vi "Create.vi"(0 "vi reference":refnum<vi>, 5 "Ctrl Sequences":string[](array[string]), 11 "error in (no error)":errorcluster) -> (4 "vi reference out":refnum<vi>, 6 "Connector Pane Type":T1, 15 "error out":errorcluster)   [LabVIEW 2018, in "NISAST VI Scripting.lvlib" / "VI.lvlib" / "Connector.lvlib"]
uses:
  Connector.lvlib
  Front Panel/Attribute/Connector Pane Type.ctl
  Front Panel/Front Panel.lvlib
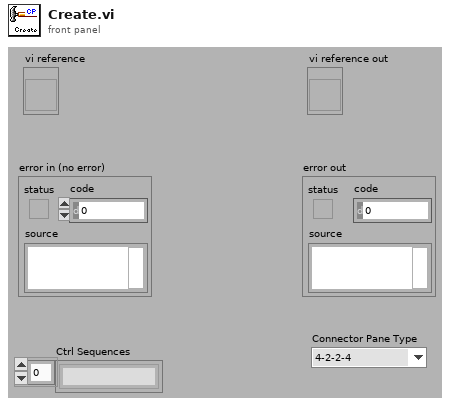
[diagram p1: front panel]
types:
  T1 = typedef "NISAST VI Scripting.lvlib/VI.lvlib/Front Panel.lvlib/Connector Pane Type.ctl" = enum16{"4-2-2-4", "5-2-2-2-5", "Others"}
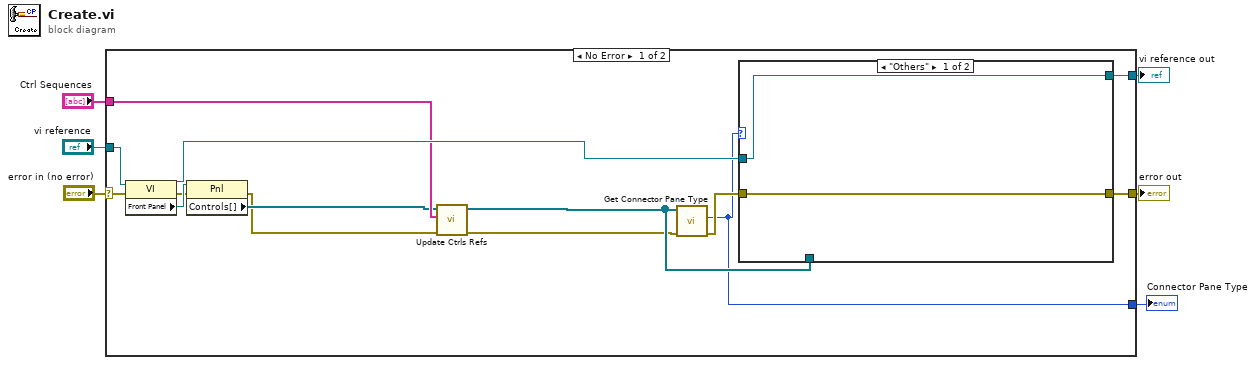
[diagram p0: block diagram]
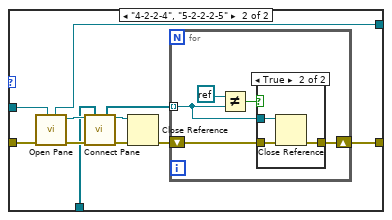
[diagram p2: hidden frame]
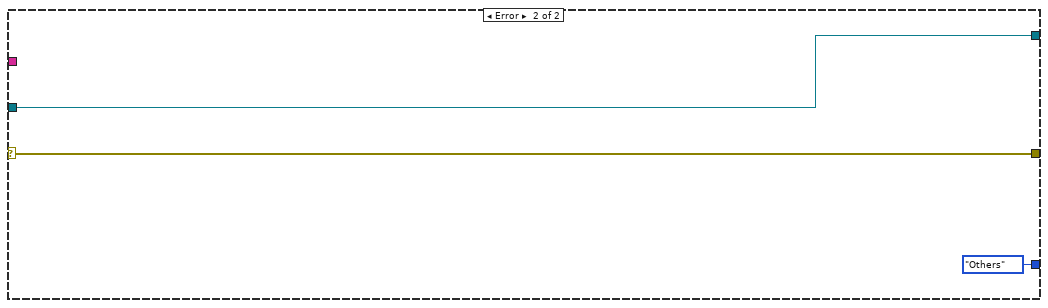
[diagram p4: hidden frame]
diagram:
  n1 = case shown="No Error" "error in (no error)" {
    selector: "error in (no error)" -> [w17 w45]
    tunnel: [w15 w45] -> w4
    tunnel: "vi reference" -> [w18 w44]
    tunnel: [w14 w44] -> w3
    tunnel: "Ctrl Sequences" -> [w13 _]
    tunnel: [w7 Connector_Pane_Type."Others" ("Connector Pane Type")] -> w1
    frame No Error {
      n2 = property class="VI"(reference=w18, error in=w17) -> (reference out=w16:refnum<vi>, error out=w19:errorcluster, "Front Panel"=w20:refnum<vi>)
      n3 = property class="Pnl"(reference=w20, error in=w19) -> (error out=w11:errorcluster, "Controls[]"=w12:refnum<vi>[])  [unwired: 1 out]
      n4 = call "Update Ctrls Refs.vi"("error in"=w11, "Ctrl Sequences"=w13, "Controls[] in"=w12) -> ("error out"=w9:errorcluster, "Controls[] out"=w10:refnum<vi>[])  [unwired: 7 out]
      n5 = call "Get Connector Pane Type.vi"("error in (no error)"=w9, "Controls[]"=w10) -> ("error out"=w8:errorcluster, "Connector Pane Type"=w7:T1)  [unwired: 7 out]
      n6 = case shown="\"Others\"" w7 {
        tunnel: w16 -> [w22 w29]
        tunnel: [w21 w26] -> w15
        tunnel: [w22 w25] -> w14
        tunnel: w10 -> [_ w24]
        tunnel: w8 -> [w21 w23]
        frame "Others" {
        }
        frame "4-2-2-4", "5-2-2-2-5" {
          n7 = call "Open Pane.vi"("vi refnum"=w29, "error in"=w23) -> ("error out"=w30:errorcluster, "connect pane"=w33:refnum<vi>, "vi refnum out"=w25:refnum<vi>)  [unwired: 7 out]
          n8 = call "Connect Pane.vi"("connect pane"=w33, "Controls[]"=w24, "error in"=w30) -> ("Controls[] output"=w27:refnum<vi>[], "connect pane out"=w32:refnum<vi>, "error out"=w31:errorcluster)  [unwired: 10 out]
          n9 = Close Reference(reference=w32, error in (no error)=w31) -> (error out=w28:errorcluster)
          n10 = for {
            shift-right: [w37] -> w26
            shift-left: w28 -> [w38]
            tunnel: w27 -> [w35] mode=indexing
            n11 = Not Equal?(x=refnum<k0> refnum, y=w35) -> (x != y?=w34:bool)
            n12 = case shown="True" w34 {
              tunnel: w38 -> [w39 w42]
              tunnel: [w39 w41] -> w37
              tunnel: w35 -> [_ w40]
              frame False {
              }
              frame True {
                n13 = Close Reference(reference=w40, error in (no error)=w42) -> (error out=w41:errorcluster)
              }
            }
          }
        }
      }
    }
    frame Error {
    }
  }
  "error out" <- w4
  "vi reference out" <- w3
  "Connector Pane Type" <- w1
